vi "Initialize.vi"(8 "error in (no error)":errorcluster, 11 "Component Configuration in":refnum<class "DSF Buffer Converter Configurations.lvclass">) -> (0 "error out":errorcluster, 3 "Component Configuration out":refnum<class "DSF Buffer Converter Configurations.lvclass">)   [LabVIEW 2017, in "DSF Core.lvlib" / "DSF Buffer Converter Configurations.lvclass"]
uses:
  DSF Buffer Converter Configurations.lvclass
  C:/Git/DSF/Core/Classes/Component Configuration/Component Configurations.lvclass
  DSF Buffer Converter Transfer Configuration.lvclass
  C:/Git/DSF/Core/Classes/Configuration/Configuration.lvclass
  Classes/Component Configuration/Component Configurations.lvclass
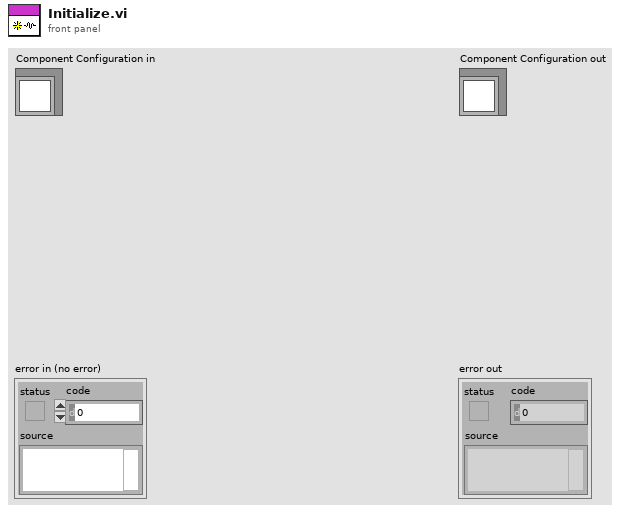
[diagram p1: front panel]
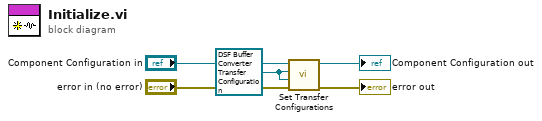
[diagram p0: block diagram]
diagram:
  w1 = refnum<class "DSF Buffer Converter Transfer Configuration.lvclass"> refnum ("DSF Core.lvlib:DSF Buffer Converter Transfer Configuration.lvclass")
  n1 = call "Set Transfer Configurations.vi"("error in (no error)"="error in (no error)", "Tx Transfer Configuration"=w1, "Rx Transfer Configuration"=w1, "Component Configuration in"="Component Configuration in") -> ("error out"=→"error out":errorcluster, "Component Configuration out"=→"Component Configuration out":refnum<class "DSF Buffer Converter Configurations.lvclass">)  [unwired: 6 in]
